vi "Stop Displacement Sensor.vi"(8 "error in (no error)":errorcluster, 11 "Model in":refnum<class "Model.lvclass">) -> (0 "error out":errorcluster, 3 "Model out":refnum<class "Model.lvclass">)   [LabVIEW 2016, in "Model.lvclass"]
uses:
  Model.lvclass
  Model.lvclass/Model.ctl
  common_serialprotocols/SerialProtocol/SerialReal/SerialReal.lvclass
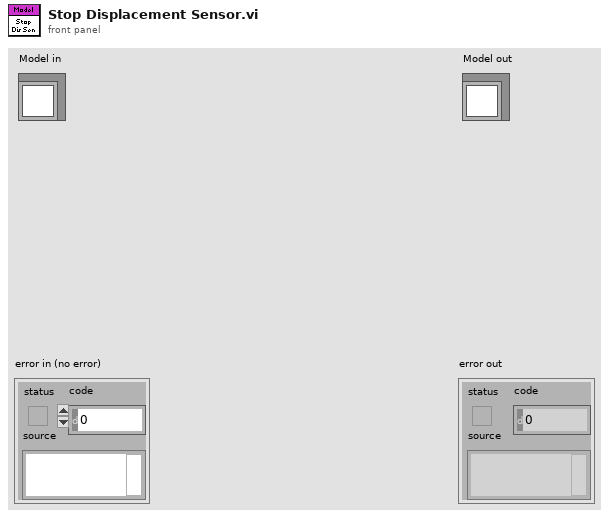
[diagram p1: front panel]
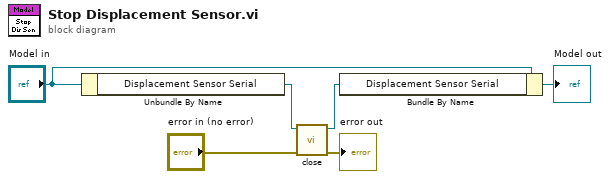
[diagram p0: block diagram]
diagram:
  n1 = Unbundle By Name("Model in") -> ("Displacement Sensor Serial"=w6:refnum<class "SerialReal.lvclass">)
  n2 = call-dynamic "close.vi"("error in (no error)"="error in (no error)", "SerialReal in"=w6) -> ("error out"=→"error out":errorcluster, "SerialReal out"=w5:refnum<class "SerialReal.lvclass">)  [unwired: 8 in]
  n3 = Bundle By Name(cluster="Model in", "Displacement Sensor Serial"=w5) -> (→"Model out":refnum<class "Model.lvclass">)
